vi "UTIL_CalLevel.vi"(9 "Key is In?":bool, 10 "Cal Coef in":T1={"M"=0.99962, "B"=9.62052, "Mc"=0.9779951100244498, "Bc"=8.5, "LMe"=8.4}, 11 "Input":dbl) -> (2 "PVc":dbl=9.622457579462102, 3 "PVs":dbl)   [LabVIEW 2024]
uses:
  Control Definitions/Def CalCoef.ctl
panel:
  # "0.99962\n9.62052"
  # "-0.999664"
  # "9.61922"
  # "TRUE if Input is Keyances Sensor\nFALSL if Input is Level Slider"
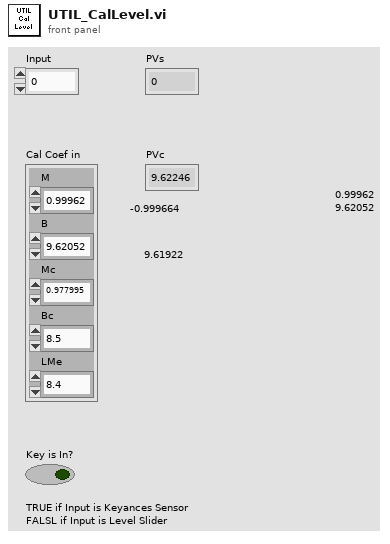
[diagram p1: front panel]
types:
  T1 = typedef "Def CalCoef.ctl" = cluster{"M":dbl, "B":dbl, "Mc":dbl, "Bc":dbl, "LMe":dbl}
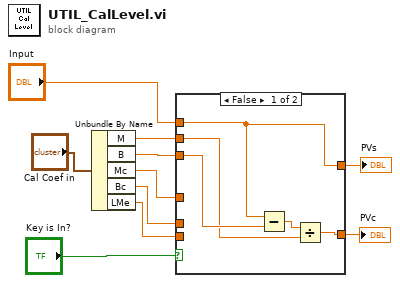
[diagram p0: block diagram]
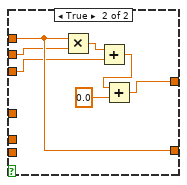
[diagram p2: hidden frame]
diagram:
  n1 = Unbundle By Name("Cal Coef in") -> ("M"=w1:dbl, "B"=w7:dbl, "Mc"=w5:dbl, "Bc"=w4:dbl, "LMe"=w6:dbl)
  n2 = case shown="False" "Key is In?" {
    tunnel: "Input" -> [w11 w21]
    tunnel: w4 -> [_ _]
    tunnel: w5 -> [_ _]
    tunnel: w6 -> [_ _]
    tunnel: w1 -> [w13 w20]
    tunnel: w7 -> [w15 w19]
    tunnel: [w11 w17] -> w8
    tunnel: [w12 w21] -> w9
    frame False {
      n3 = Subtract(x=w11, y=w15) -> (x-y=w14:dbl)
      n4 = Divide(x=w14, y=w13) -> (x/y=w12:dbl)
    }
    frame True {
      n5 = Multiply(x=w21, y=w20) -> (x*y=w22:dbl)
      n6 = Add(x=w22, y=w19) -> (x+y=w18:dbl)
      n7 = Add(x=w18, y=0.0) -> (x+y=w17:dbl)
    }
  }
  "PVs" <- w8
  "PVc" <- w9
